vi "Read Relays.vi"(8 "error in (no error)":errorcluster, 11 "Switch Action Processor in":refnum<class "Switch Action Processor.lvclass">) -> (0 "error out":errorcluster, 2 "Relays":refnum<class "Relay.lvclass">[](array[class]))   [LabVIEW 2015, in "SLSC Switch.lvlib" / "Switch Action Processor.lvclass"]
uses:
  Switch Action Processor.lvclass
  Relay/Relay.lvclass
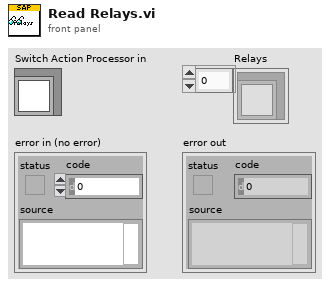
[diagram p1: front panel]
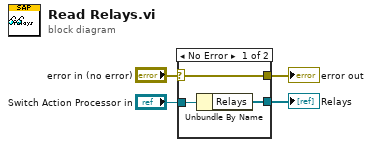
[diagram p0: block diagram]
diagram:
  n1 = case shown="No Error" "error in (no error)" {
    selector: "error in (no error)" -> [w7 w8]
    tunnel: [w7 w8] -> w3
    tunnel: "Switch Action Processor in" -> [w6 _]
    tunnel: [w5 _] -> w1
    frame No Error {
      n2 = Unbundle By Name(w6) -> ("Relays"=w5:refnum<class "Relay.lvclass">[])
    }
    frame Error {
    }
  }
  "error out" <- w3
  "Relays" <- w1
